vi "BSJShipPackage.vi"(8 "error in":errorcluster caption="错误输入", 11 "包装箱条码":string) -> (0 "error out":errorcluster caption="错误输出", 3 "OK？":bool)   [LabVIEW 2013]
panel:
  out "元素":string
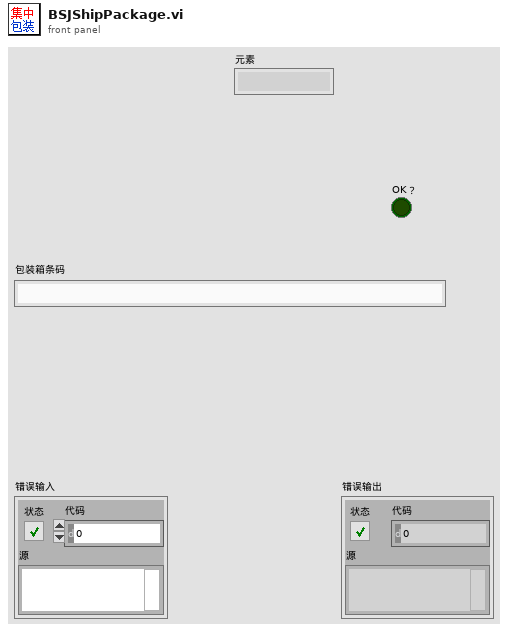
[diagram p1: front panel]
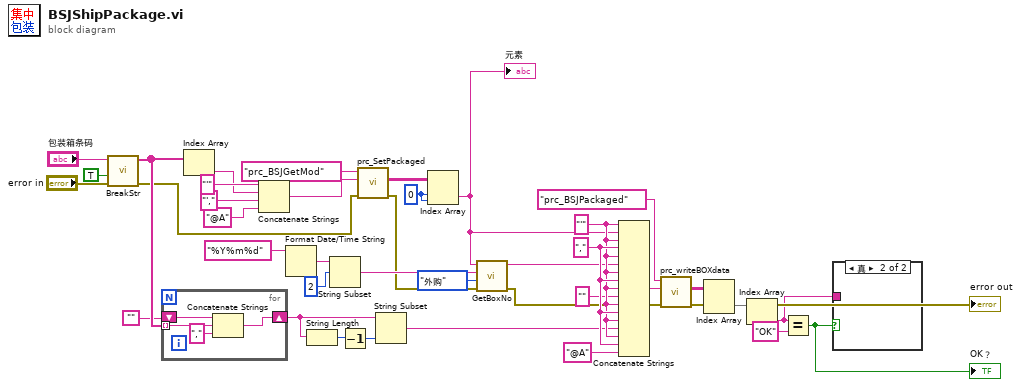
[diagram p0: block diagram]
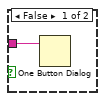
[diagram p2: hidden frame]
diagram:
  w21 = 0
  w39 = ","
  w36 = "'"
  n1 = call "BreakStr.vi"("error in"="error in", "外购？"=TRUE, "StrIn"="包装箱条码") -> ("error out"=w7:errorcluster, "ArrayOut"=w16:string[])  [unwired: 7 in]
  n2 = for {
    shift-right: [w42] -> w14
    shift-left: "" -> [w43]
    tunnel: w16 -> [w40] mode=indexing
    n3 = Concatenate Strings(w43, w40, ",") -> (w42:string)
  }
  n4 = Index Array(array=w16) -> (element=w26:string)  [unwired: 1 in]
  n5 = Concatenate Strings("'", w26, "',", "@A" ("字符串")) -> (w23:string)
  n6 = Format Date/Time String(time format string (%c)="%Y%m%d" ("时间格式字符串(%c)")) -> (date/time string=w35:string)  [unwired: 2 in]
  n7 = String Length(string=w14) -> (length=w13:i32)
  n8 = String Subset(string=w35, offset (0)=2 ("偏移量(0)")) -> (substring=w33:string)  [unwired: 1 in]
  n9 = Decrement(x=w13) -> (x-1=w12:i32)
  n10 = call "prc_SetPackaged.vi"("error in"=w7, "string"=w23, "SQL query"="prc_BSJGetMod") -> ("error out"=w20:errorcluster, "Array"=w22:string[][])  [unwired: 7 in]
  n11 = String Subset(string=w14, length (rest)=w12) -> (substring=w11:string)  [unwired: 1 in]
  n12 = Index Array(array=w22, index (row)=w21, index (col)=w21) -> (element=w19:string)
  "元素" <- w19
  n13 = call "GetBoxNo.vi"("error in"=w20, "种类"=enum16{"自产", "外购"}."外购", "TimeStr"=w33, "Model"=w19) -> ("error out"=w9:errorcluster, "BoxNo"=w32:string)  [unwired: 6 in]
  n14 = Concatenate Strings(w36, w19, w36, w39, w36, w32, w36, w39, w36, "", w36, w39, w36, w11, w36, w39, "@A" ("字符串")) -> (w38:string)
  n15 = call "prc_writeBOXdata.vi"("error in"=w9, "string"=w38, "Process"="prc_BSJPackaged") -> ("error out"=→"error out":errorcluster, "Array"=w37:string[][])  [unwired: 7 in]
  n16 = Index Array(array=w37) -> (element=w30:string[])  [unwired: 2 in]
  n17 = Index Array(array=w30) -> (element=w4:string)  [unwired: 1 in]
  n18 = Equal?(x=w4, y="OK") -> (x = y?=w5:bool)
  "OK？" <- w5
  n19 = case shown="真" w5 {
    tunnel: w4 -> [w44 _]
    frame False {
      n20 = One Button Dialog(message=w44) -> ()  [unwired: 1 in, 1 out]
    }
    frame True {
    }
  }
